vi "Icai 105 - Simultry1_triggering adjustment.vi"() -> ()   [LabVIEW 2010]
uses:
  <vilib>/Utility/error.llb/DialogType.ctl
  <vilib>/DAQmx/write.llb/DAQmx Write (Analog DBL 1Chan 1Samp).vi
  <vilib>/DAQmx/write.llb/DAQmx Write (Digital 1D Bool 1Chan 1Samp).vi
  <vilib>/DAQmx/write.llb/DAQmx Write (Analog 1D Wfm NChan NSamp).vi
  <vilib>/DAQmx/write.llb/DAQmx Write (Analog Wfm 1Chan NSamp).vi
  <vilib>/DAQmx/create/channels.llb/DAQmx Create Channel (AO-Voltage-Basic).vi
  <vilib>/daqmx/miscellaneous.llb/DAQmx Fill In Error Info.vi
  <vilib>/Waveform/WDTOps.llb/WDT Append Waveforms DBL.vi
  <vilib>/measure/matone.llb/Extract Single Tone Information 1 Chan.vi
  <vilib>/DAQmx/create/channels.llb/DAQmx Create Channel (DO-Digital Output).vi
  <vilib>/DAQmx/configure/timing.llb/DAQmx Timing (Sample Clock).vi
  <vilib>/DAQmx/configure/trigger.llb/DAQmx Start Trigger (Digital Edge).vi
  <vilib>/measure/NI_MABase.lvlib
  <vilib>/measure/NI_MAPro.lvlib
  Program Files/National Instruments/LabVIEW 2010/resource/objmgr/daqmx.rc
panel:
  out "number of samples written per channel":u32
  in  "rate":dbl=10000000.0
  out "detected frequency 2":dbl format="%.6p"
  out "SampClk.Timebase.Rate":dbl format="%^#_10g"
  in  "Freq Scale Factor":dbl=1.0 format="%#_12g"
  out "detected frequency":dbl format="%.6p"
  out "signal out":waveform(dbl)(graph)
  in  "lines":tag="Dev1/port0/line3"
  in  "Rising Logic Output Chan":tag="Dev1/ao2"
  in  "Mod Duration ms":i32=300
  in  "Samples (1Ms/s)":i32=700000
  out "min value":dbl
  in  "Falling Logic Output Chan":tag="Dev1/ao1"
  in  "FM Waveform Channel":tag="Dev1/ao3"
  out "error out":errorcluster caption="error out (DAQ)"
  out "Mod":dbl=118572.0
  out "Numeric 2":dbl=3900000.0 format="%#_7g"
  out "Numeric":dbl=3900000.0 format="%#_7g"
  in  "Pre-Trig Samples":ext=100.0 format="%.2f"
  out "?":dbl=579698.7113293351 format="%#_6f"
  out "#s":dbl=39524.02451426849
  in  "Time int":i32=1000
  in  "Sensitivity":u16(ring)=14 items=["2 nV/fA", "5 nV/fA", "10 nV/fA", "20 nV/fA", "50 nV/fA", "100 nV/fA", "200 nV/fA", "500 nV/fA", "1 uV/pA", "2 uV/pA", "5 uV/pA", "10 uV/pA", "20 uV/pA", "50 uV/pA", "100 uV/pA", "200 uV/pA", "500 uV/pA", "1 mV/nA", "2 mV/nA", "5 mV/nA", "10 mV/nA", "20 mV/nA", "50 mV/nA", "100 mV/nA", "200 mV/nA", "500 mV/nA", "1 V/uA"]
  in  "Detection Bandwidth":u16(ring)=7 items=["10 us/ 25 kHz", "30 us /8.33 kHz", "100 us/ 2.50 kHz", "300 us/ 833 Hz", "1 ms /250 Hz", "3 ms /83.3 Hz", "10 ms/ 25 Hz", "30 ms/ 8.33 Hz", "100 ms/ 2.50 Hz", "300 ms/ 0.833 Hz ", "1 s/ 0.250 Hz", "3 s/ 0.0833 Hz", "10 s/0.025 Hz"]
  in  "SR 830 GPIB Address":i32=8
  in  "Freq 2":dbl=2448.0 format="%_7g"
  out "Iterat #":dbl=10.0
  in  "Iteration":dbl=17.0
  in  "stop 2":bool
  in  "pulse":bool=TRUE
  in  "Start":ext=0.05
  out "?":waveform(dbl)[](graph)
  in  "amplitude 2":dbl=0.25 format="%0.2p"
  in  "?":T1(ring)=enum."Triangle Wave"
  in  "phase 2":dbl format="%.2p"
  in  "Offset 2":dbl=-0.0 format="%#_6p"
  in  "frequency 4":dbl=100.0 format="%0.2p"
  in  "?":T1(ring)=enum."Triangle Wave"
  in  "offset 4":dbl=-1.0 format="%0.2p"
  in  "phase 4":dbl=90.0 format="%.2p"
  in  "amplitude 4":dbl=1.0 format="%0.2p"
  in  "frequency 1":dbl=100.0 format="%0.2p"
  in  "amplitude 1":dbl=1.0 format="%0.2p"
  in  "sampling info 1":cluster{"Fs":dbl, "#s":dbl}={"Fs"=1000000.0, "#s"=2500.0} {"Fs" format="%.2p"}
  in  "?":T1(ring)=enum."Triangle Wave"
  in  "phase 1":dbl=-90.0 format="%.2p"
  in  "Offset 1":dbl format="%#_6p"
  in  "iterat":dbl
  out "CW":dbl=123571.0
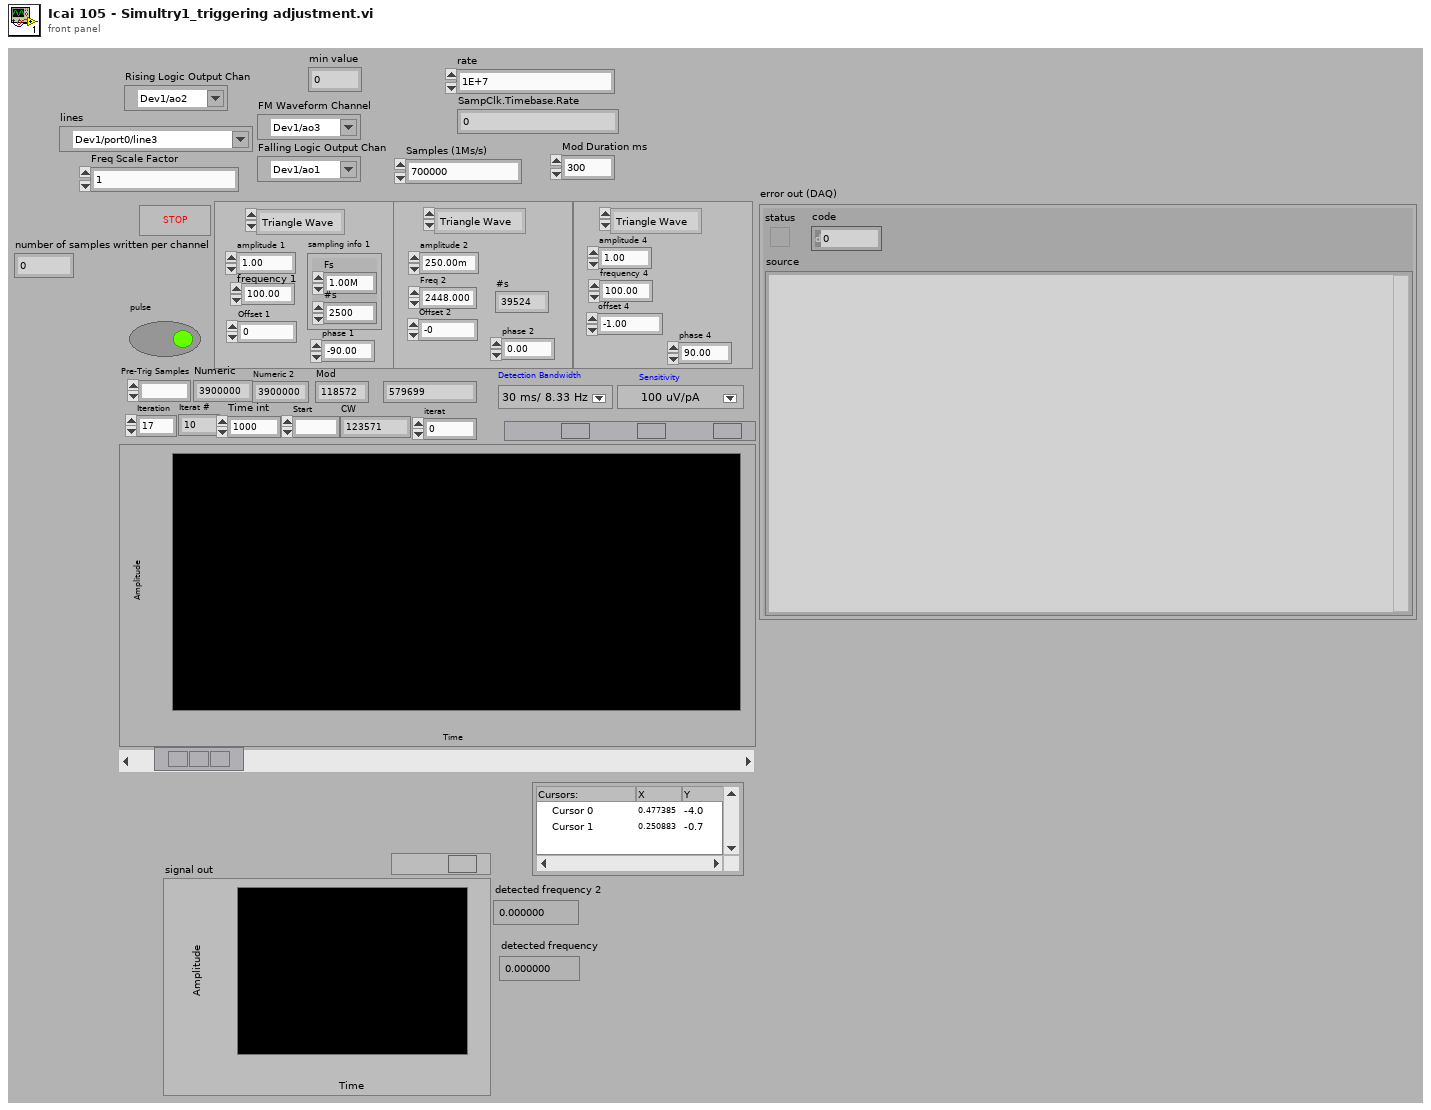
[diagram p1: front panel]
types:
  T1 = enum16{"Sine Wave", "Triangle Wave", "Square Wave", "Sawtooth Wave"}
  T2 = typedef "DialogType.ctl" = u16
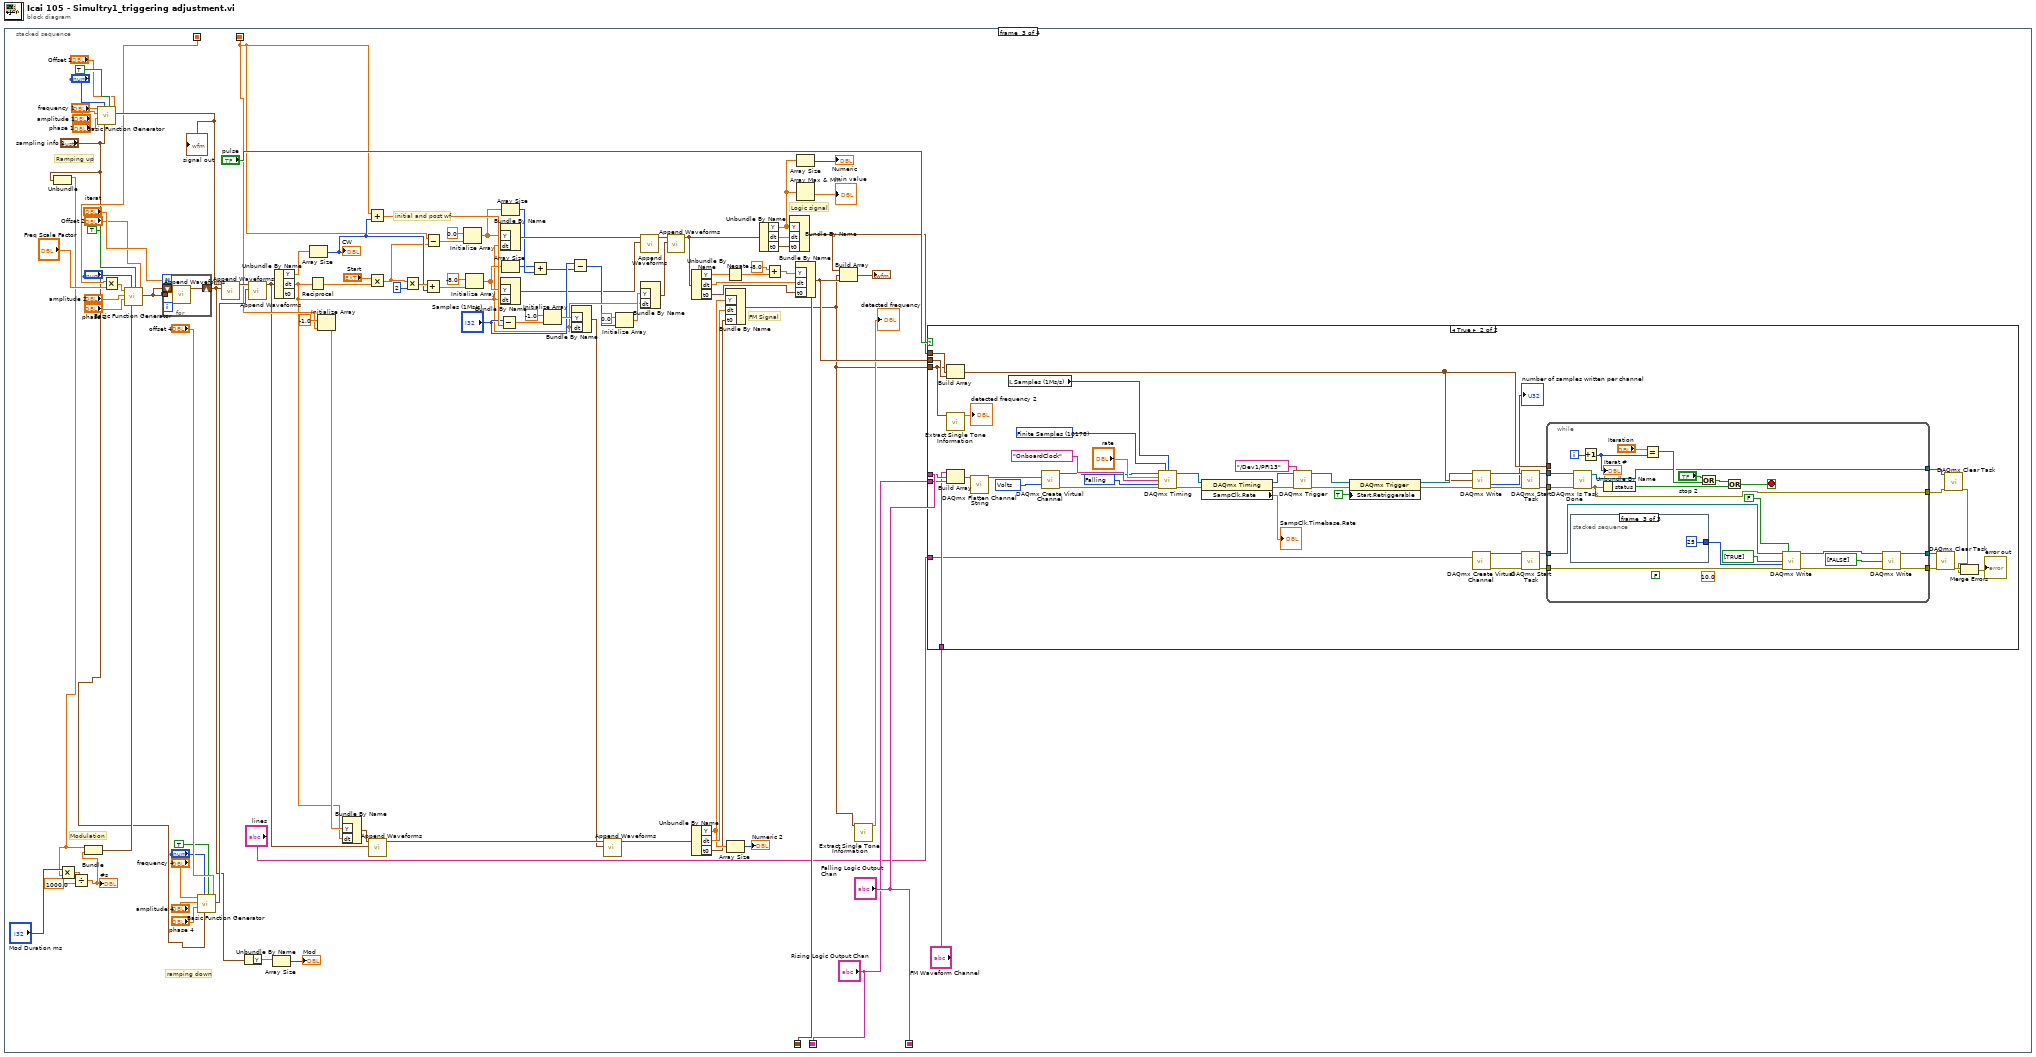
[diagram p0: block diagram]
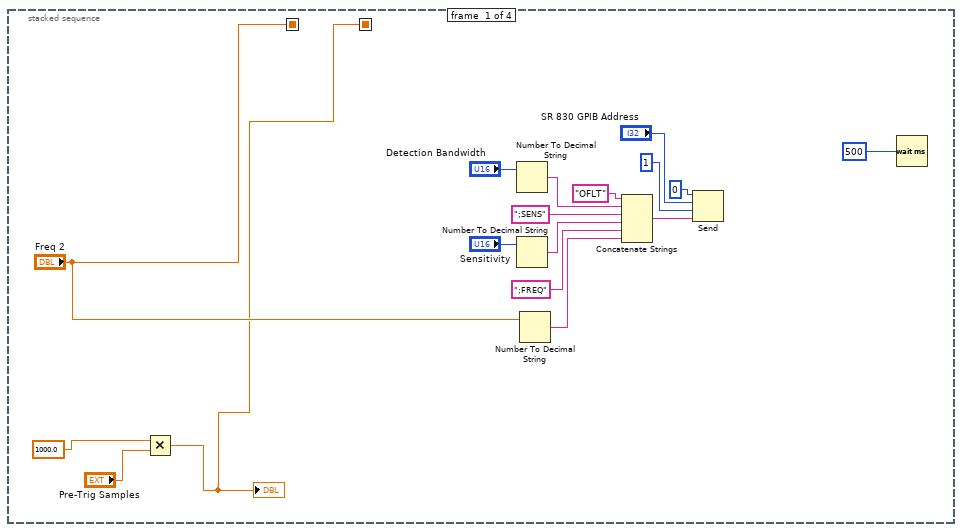
[diagram p2: hidden frame]
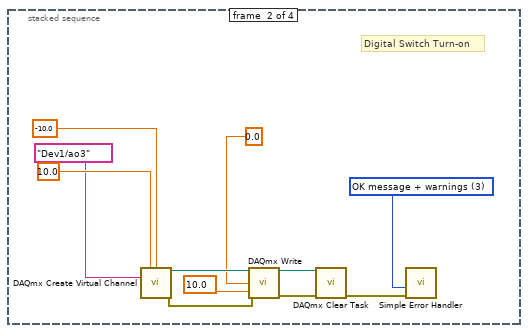
[diagram p3: hidden frame]
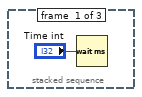
[diagram p5: hidden frame]
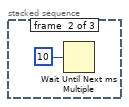
[diagram p6: hidden frame]
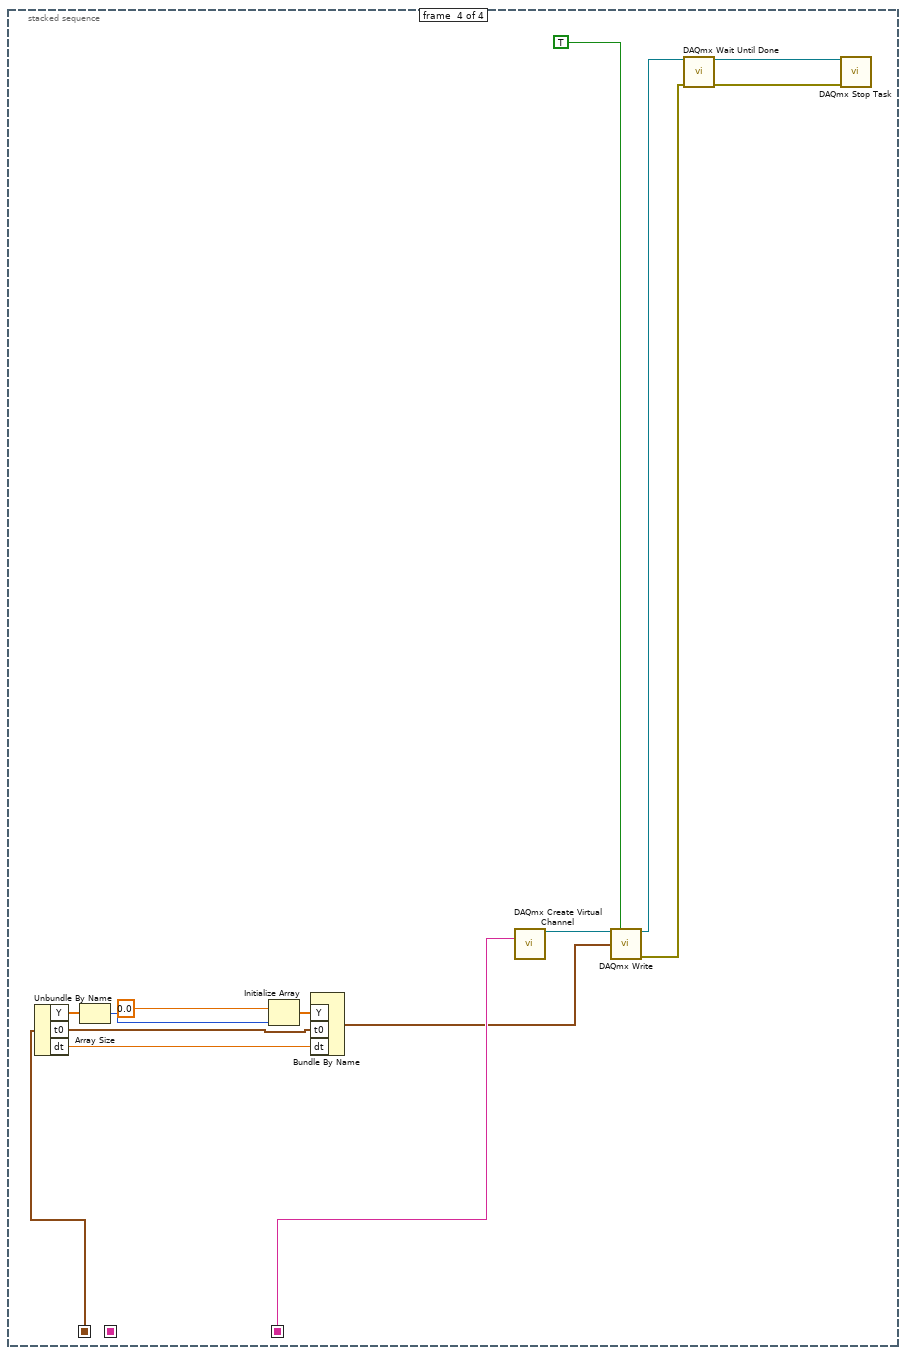
[diagram p7: hidden frame]
diagram:
  n1 = stacked-sequence {
    seq-local: ["Freq 2" _ _ _] -> [_ _ w34 _]
    seq-local: [w1 _ _ _] -> [_ _ w69 _]
    seq-local: [_ _ "Falling Logic Output Chan" _] -> [_ _ _ w202]
    seq-local: [_ _ "Rising Logic Output Chan" _] -> [_ _ _ _]
    seq-local: [_ _ w49 _] -> [_ _ _ w210]
    frame #0 {
      n2 = Multiply(x=1000.0 ("Fs 2"), y="Pre-Trig Samples") -> (x*y=w1:ext)
      "?" <- w1
      n3 = Number To Decimal String(number="Detection Bandwidth") -> (decimal integer string=w16:string)  [unwired: 1 out]
      n4 = Number To Decimal String(number="Sensitivity") -> (decimal integer string=w14:string)  [unwired: 1 out]
      n5 = Number To Decimal String(number="Freq 2") -> (decimal integer string=w5:string)  [unwired: 1 out]
      n6 = Concatenate Strings("OFLT", w16, ";SENS", w14, ";FREQ" ("string"), w5) -> (w13:string)
      n7 = Send(0:0 ("bus"), 2:"SR 830 GPIB Address", 3:i16 1 ("mode"), 5:w13) -> ()  [unwired: 1 in, 3 out]
      n8 = Wait (ms)(milliseconds to wait=500) -> ()  [unwired: 1 out]
    }
    frame #1 {
      w21 = T2 3 items=["no dialog", "OK message", "continue or stop message", "OK message + warnings", "continue/stop + warnings"] ("type of dialog (OK msg:1)")
      # "Digital Switch Turn-on"
      n9 = call-poly <vilib>:"DAQmx Create Virtual Channel.vi"("maximum value"=10.0 ("Maximum Value"), "minimum value"=-10.0 ("Minimum Value"), "physical channels"=tag "Dev1/ao3" ("Physical Channel")) -> ("task out"=w24:refnum<k21>, "error out"=w25:errorcluster)  [unwired: 6 in, 5 out]
      n10 = call-poly <vilib>:"DAQmx Write.vi"("task/channels in"=w24, "data"=0.0 ("Voltage Output"), "timeout"=10.0, "error in"=w25) -> ("task out"=w19:refnum<k21>, "error out"=w20:errorcluster)  [unwired: 1 in, 9 out]
      n11 = call <vilib>:"DAQmx Clear Task.vi"("task in"=w19, "error in"=w20) -> ("error out"=w18:errorcluster)  [unwired: 13 out]
      n12 = call <vilib>:"Simple Error Handler.vi"("type of dialog (OK msg:1)"=w21, "error in (no error)"=w18) -> ()  [unwired: 8 out]
    }
    frame #2 {
      # "initial and post wf"
      # "FM Signal"
      # "Logic signal"
      # "Ramping up"
      # "ramping down"
      # "Modulation"
      n13 = Unbundle("sampling info 1") -> ("Fs"=w31:dbl)  [unwired: 1 out]
      n14 = Multiply(x="Mod Duration ms", y=w31) -> (x*y=w41:dbl)
      n15 = Divide(x=w41, y=1000.0) -> (x/y=w39:dbl)
      "#s" <- w39
      n16 = Bundle("Fs"=w31, w39) -> (w73:cluster{"Fs":dbl, dbl})  [unwired: 1 out]
      n17 = call <vilib>:"Basic Function Generator.vi"("offset"="Offset 1", "reset signal"=TRUE, "sampling info"="sampling info 1", "signal type"="?", "phase"="phase 1", "amplitude"="amplitude 1", "frequency"="frequency 1") -> ("signal out"=w107:waveform(dbl))  [unwired: 2 in, 2 out]
      "signal out" <- w107
      n18 = Multiply(x=w34, y="Freq Scale Factor") -> (x*y=w33:dbl)
      n19 = call <vilib>:"Basic Function Generator.vi"("offset"="Offset 2", "reset signal"=TRUE, "sampling info"=w73, "signal type"="?", "phase"="phase 2", "amplitude"="amplitude 2", "frequency"=w33) -> ("signal out"=w37:waveform(dbl))  [unwired: 2 in, 2 out]
      n20 = for {
        N: "iterat" -> [_]
        shift-right: [w200] -> w62
        shift-left: w37 -> [w198]
        tunnel: w37 -> [w199]
        n21 = call-poly <vilib>:"Append Waveforms.vi"("waveform B"=w199, "waveform A"=w198) -> ("waveform out"=w200:waveform(dbl))  [unwired: 1 in, 8 out]
      }
      n22 = call <vilib>:"Basic Function Generator.vi"("offset"="offset 4", "reset signal"=TRUE, "sampling info"="sampling info 1", "signal type"="?", "phase"="phase 4", "amplitude"="amplitude 4", "frequency"="frequency 4") -> ("signal out"=w112:waveform(dbl))  [unwired: 2 in, 2 out]
      n23 = call-poly <vilib>:"Append Waveforms.vi"("waveform B"=w62, "waveform A"=w107) -> ("waveform out"=w106:waveform(dbl))  [unwired: 1 in, 8 out]
      n24 = Unbundle By Name(w62) -> ("Y"=w63:dbl[])
      n25 = call-poly <vilib>:"Append Waveforms.vi"("waveform B"=w112, "waveform A"=w106) -> ("waveform out"=w45:waveform(dbl))  [unwired: 1 in, 8 out]
      n26 = Array Size(array=w63) -> (size(s)=→"Mod":i32)
      n27 = Unbundle By Name(w45) -> ("Y"=w108:dbl[], "dt"=w68:dbl)  [unwired: 1 out]
      n28 = Reciprocal(x=w68) -> (1/x=w70:dbl)
      n29 = Array Size(array=w108) -> (size(s)=w90:i32)
      "CW" <- w90
      n30 = Initialize Array(-1.0 ("DC level"), w69) -> (w97:dbl[])
      n31 = Bundle By Name("Y"=w97, "dt"=w68) -> (w110:waveform(dbl))  [unwired: 1 out]
      n32 = Add(x=w69, y=w90) -> (x+y=w95:ext)
      n33 = Multiply(x="Start", y=w70) -> (x*y=w83:ext)
      n34 = call-poly <vilib>:"Append Waveforms.vi"("waveform B"=w45, "waveform A"=w110) -> ("waveform out"=w111:waveform(dbl))  [unwired: 1 in, 8 out]
      n35 = Multiply(x=w83, y=2) -> (x*y=w91:ext)
      n36 = Add(x=w91, y=w90) -> (x+y=w72:ext)
      n37 = Subtract(x=w69, y=w83) -> (x-y=w84:ext)
      n38 = Initialize Array(0.0 ("Trigger down"), w84) -> (w82:dbl[])
      n39 = Initialize Array(-8.0 ("Trigger up"), w72) -> (w81:dbl[])
      n40 = Subtract(x="Samples (1Ms/s)", y=w95) -> (x-y=w94:ext)
      n41 = Bundle By Name("Y"=w82, "dt"=w68) -> (w86:waveform(dbl))  [unwired: 1 out]
      n42 = Bundle By Name("Y"=w81, "dt"=w68) -> (w43:waveform(dbl))  [unwired: 1 out]
      n43 = Array Size(array=w82) -> (size(s)=w80:i32)
      n44 = Array Size(array=w81) -> (size(s)=w79:i32)
      n45 = Add(x=w79, y=w80) -> (x+y=w78:i32)
      n46 = Initialize Array(-1.0 ("DC level"), w94) -> (w93:dbl[])
      n47 = Subtract(x="Samples (1Ms/s)", y=w78) -> (x-y=w44:i32)
      n48 = Bundle By Name("Y"=w93, "dt"=w68) -> (w92:waveform(dbl))  [unwired: 1 out]
      n49 = call-poly <vilib>:"Append Waveforms.vi"("waveform B"=w92, "waveform A"=w111) -> ("waveform out"=w100:waveform(dbl))  [unwired: 1 in, 8 out]
      n50 = Initialize Array(0.0 ("Trigger down"), w44) -> (w87:dbl[])
      n51 = Bundle By Name("Y"=w87, "dt"=w68) -> (w85:waveform(dbl))  [unwired: 1 out]
      n52 = call-poly <vilib>:"Append Waveforms.vi"("waveform B"=w43, "waveform A"=w86) -> ("waveform out"=w103:waveform(dbl))  [unwired: 1 in, 8 out]
      n53 = call-poly <vilib>:"Append Waveforms.vi"("waveform B"=w85, "waveform A"=w103) -> ("waveform out"=w60:waveform(dbl))  [unwired: 1 in, 8 out]
      n54 = Unbundle By Name(w60) -> ("Y"=w59:dbl[], "dt"=w54:dbl, "t0"=w55:timestamp)
      n55 = Unbundle By Name(w100) -> ("Y"=w65:dbl[], "dt"=w99:dbl, "t0"=w42:timestamp)
      n56 = Bundle By Name("Y"=w65, "dt"=w99, "t0"=w42) -> (w35:waveform(dbl))  [unwired: 1 out]
      n57 = Negate(x=w59) -> (-x=w57:dbl[])
      n58 = Array Size(array=w65) -> (size(s)=→"Numeric 2":i32)
      n59 = Unbundle By Name(w60) -> ("Y"=w61:dbl[], "dt"=w101:dbl, "t0"=w56:timestamp)
      n60 = Add(x=-8.0, y=w57) -> (x+y=w53:dbl[])
      n61 = Bundle By Name("Y"=w61, "dt"=w101, "t0"=w56) -> (w48:waveform(dbl))  [unwired: 1 out]
      n62 = Bundle By Name("Y"=w53, "dt"=w54, "t0"=w55) -> (w49:waveform(dbl))  [unwired: 1 out]
      n63 = Array Size(array=w61) -> (size(s)=→"Numeric":i32)
      n64 = Array Max & Min(array=w61) -> (min value=→"min value":dbl)  [unwired: 3 out]
      n65 = Build Array(w48, w35, w49) -> (→"?":waveform(dbl)[])
      n66 = call-poly <vilib>:"Extract Single Tone Information.vi"("time signal in"=w35) -> ("detected frequency"=→"detected frequency":dbl)  [unwired: 5 in, 5 out]
      n67 = case shown="True" "pulse" {
        tunnel: w35 -> [_ w152]
        tunnel: w48 -> [_ w169]
        tunnel: w49 -> [_ w154]
        tunnel: "Falling Logic Output Chan" -> [_ w150]
        tunnel: "Rising Logic Output Chan" -> [_ w149]
        tunnel: "lines" -> [_ w128]
        tunnel: "FM Waveform Channel" -> [_ w145]
        frame False {
        }
        frame True {
          w158 = 10348 items=["Volts"=10348, "From Custom Scale"=10065] ("units")
          w170 = 10178 items=["Finite Samples"=10178, "Continuous Samples"=10123, "Hardware Timed Single Point"=12522] ("sample mode")
          w171 = 10171 items=["Rising"=10280, "Falling"=10171] ("active edge")
          n68 = Build Array(w152, w169, w154) -> (w133:waveform(dbl)[])
          n69 = call-poly <vilib>:"Extract Single Tone Information.vi"("time signal in"=w152) -> ("detected frequency"=→"detected frequency 2":dbl)  [unwired: 5 in, 5 out]
          n70 = Build Array(w145, w150, w149) -> (w151:tag[])
          n71 = call <vilib>:"DAQmx Flatten Channel String.vi"("names in"=w151) -> ("names out"=w146:string)  [unwired: 13 in, 1 out]
          n72 = local read "Samples (1Ms/s)"() -> (w165:i32)
          n73 = call-poly <vilib>:"DAQmx Create Virtual Channel.vi"("physical channels"=w146, "units"=w158) -> ("task out"=w148:refnum<k21>, "error out"=w147:errorcluster)  [unwired: 12 in]
          n74 = call-poly <vilib>:"DAQmx Timing.vi"("task/channels in"=w148, "sample mode"=w170, "samples per channel"=w165, "rate"="rate", "source"=tag "OnboardClock", "active edge"=w171, "error in"=w147) -> ("task out"=w157:refnum<k21>, "error out"=w156:errorcluster)  [unwired: 7 in]
          n75 = property class="DAQmx Timing"(reference=w157, error in=w156) -> (reference out=w144:refnum<k21>, error out=w143:errorcluster, "SampClk.Rate"=→"SampClk.Timebase.Rate":dbl)
          n76 = call-poly <vilib>:"DAQmx Trigger.vi"("task/channels in"=w144, "source"=tag "/Dev1/PFI13", "error in"=w143) -> ("task out"=w142:refnum<k21>, "error out"=w141:errorcluster)  [unwired: 11 in]
          n77 = property class="DAQmx Trigger"(reference=w142, error in=w141, "Start.Retriggerable"=TRUE) -> (reference out=w139:refnum<k21>, error out=w140:errorcluster)
          n78 = call-poly <vilib>:"DAQmx Write.vi"("task/channels in"=w139, "data"=w133, "error in"=w140) -> ("task out"=w137:refnum<k21>, "number of samples written per channel"=→"number of samples written per channel":u32, "error out"=w136:errorcluster)  [unwired: 10 in]
          n79 = call-poly <vilib>:"DAQmx Create Virtual Channel.vi"("lines"=w128) -> ("task out"=w164:refnum<k21>, "error out"=w159:errorcluster)  [unwired: 13 in]
          n80 = call <vilib>:"DAQmx Start Task.vi"("task/channels in"=w137, "error in"=w136) -> ("task out"=w135:refnum<k21>, "error out"=w134:errorcluster)  [unwired: 12 in]
          n81 = call <vilib>:"DAQmx Start Task.vi"("task/channels in"=w164, "error in"=w159) -> ("task out"=w168:refnum<k21>, "error out"=w167:errorcluster)  [unwired: 12 in]
          n82 = while {
            tunnel: w133 -> [_]
            tunnel: w168 -> [w188]
            tunnel: w167 -> [w186]
            tunnel: [w181] -> w162
            tunnel: [w180] -> w163
            tunnel: w135 -> [w176]
            tunnel: w134 -> [w175]
            tunnel: [w174] -> w131
            tunnel: [w173] -> w130
            i -> [w192]
            stop <- w178 stop-if-true
            (unwired) FALSE ("auto start")
            (unwired) 10.0 ("timeout (sec)")
            n83 = stacked-sequence {
              tunnel: [_ _ 25 ("timeout (s)")] -> w189
              frame #0 {
                n84 = Wait (ms)(milliseconds to wait="Time int") -> ()  [unwired: 1 out]
              }
              frame #1 {
                n85 = Wait Until Next ms Multiple(millisecond multiple=u32 10) -> ()  [unwired: 1 out]
              }
              frame #2 {
              }
            }
            n86 = call <vilib>:"DAQmx Is Task Done.vi"("task/channels in"=w176, "error in"=w175) -> ("task out"=w174:refnum<k21>, "error out"=w173:errorcluster)  [unwired: 11 in, 1 out]
            n87 = Increment(x=w192) -> (x+1=w190:i32)
            "Iterat #" <- w190
            n88 = Unbundle By Name(w173) -> ("status"=w177:bool)
            n89 = Equal?(x="Iteration", y=w190) -> (x = y?=w194:bool)
            n90 = Or(x="stop 2", y=w194) -> (x .or. y?=w179:bool)
            n91 = Or(x=w179, y=w177) -> (x .or. y?=w178:bool)
            n92 = call-poly <vilib>:"DAQmx Write.vi"("task/channels in"=w188, "auto start"=FALSE, "data"=bool[] [TRUE], "timeout"=w189, "error in"=w186) -> ("task out"=w184:refnum<k21>, "error out"=w182:errorcluster)  [unwired: 8 in, 1 out]
            n93 = call-poly <vilib>:"DAQmx Write.vi"("task/channels in"=w184, "data"=bool[] [FALSE], "error in"=w182) -> ("task out"=w180:refnum<k21>, "error out"=w181:errorcluster)  [unwired: 10 in, 1 out]
          }
          n94 = call <vilib>:"DAQmx Clear Task.vi"("task in"=w163, "error in"=w162) -> ("error out"=w161:errorcluster)  [unwired: 13 in]
          n95 = call <vilib>:"DAQmx Clear Task.vi"("task in"=w131, "error in"=w130) -> ("error out"=w129:errorcluster)  [unwired: 13 in]
          n96 = Merge Errors(w161, w129) -> (→"error out":errorcluster)
        }
      }
    }
    frame #3 {
      n97 = Unbundle By Name(w210) -> ("Y"=w207:dbl[], "t0"=w209:timestamp, "dt"=w208:dbl)
      n98 = Array Size(array=w207) -> (size(s)=w206:i32)
      n99 = Initialize Array(0.0 ("element"), w206) -> (w204:dbl[])
      n100 = Bundle By Name("Y"=w204, "t0"=w209, "dt"=w208) -> (w201:waveform(dbl))  [unwired: 1 in]
      n101 = call-poly <vilib>:"DAQmx Create Virtual Channel.vi"("physical channels"=w202) -> ("task out"=w203:refnum<k21>)  [unwired: 13 in, 1 out]
      n102 = call-poly <vilib>:"DAQmx Write.vi"("task/channels in"=w203, "auto start"=TRUE, "data"=w201) -> ("task out"=w211:refnum<k21>, "error out"=w214:errorcluster)  [unwired: 10 in, 1 out]
      n103 = call <vilib>:"DAQmx Wait Until Done.vi"("task/channels in"=w211, "error in"=w214) -> ("task out"=w213:refnum<k21>, "error out"=w215:errorcluster)  [unwired: 12 in]
      n104 = call <vilib>:"DAQmx Stop Task.vi"("task/channels in"=w213, "error in"=w215) -> ()  [unwired: 12 in, 2 out]
    }
  }
